vi "Send WPIN Command.vi"(0 "Serial Devices in":refnum<class "Serial Devices.lvclass">, 5 "Device":string, 7 "Puerto":u8, 9 "Pin":u8, 11 "error in":errorcluster, 12 "Valor":string) -> (4 "Serial Devices out":refnum<class "Serial Devices.lvclass">, 6 "Command":string, 10 "Expected":string, 15 "error out":errorcluster)   [LabVIEW 2019, in "Serial Devices.lvlib" / "Serial Devices.lvclass"]
uses:
  Serial Devices.lvclass
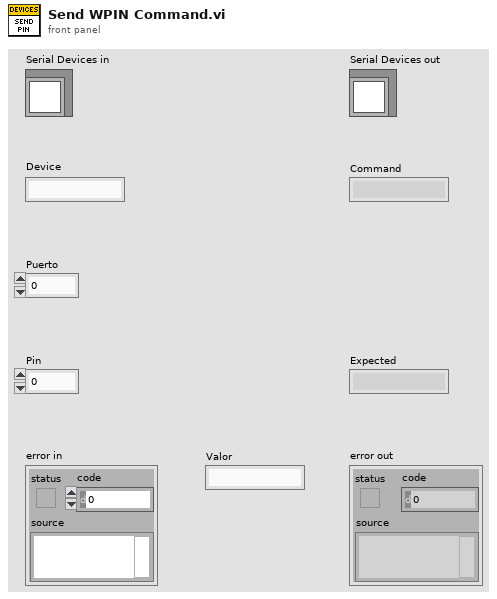
[diagram p1: front panel]
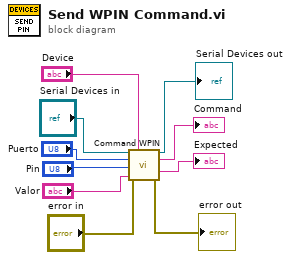
[diagram p0: block diagram]
diagram:
  n1 = call "Command WPIN.vi"("Serial Devices in"="Serial Devices in", "Device"="Device", "Puerto"="Puerto", "Pin"="Pin", "Valor"="Valor", "error in (no error)"="error in") -> ("Serial Devices out"=→"Serial Devices out":refnum<class "Serial Devices.lvclass">, "Command"=→"Command":string, "Expected"=→"Expected":string, "error out"=→"error out":errorcluster)  [unwired: 6 in]
